vi "fade.vi"(8 "Brightness":dbl, 11 "In":u32) -> (3 "Out":u32)   [LabVIEW 2016]
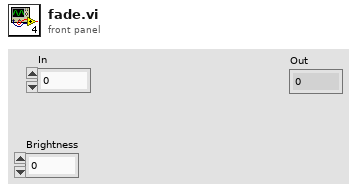
[diagram p1: front panel]
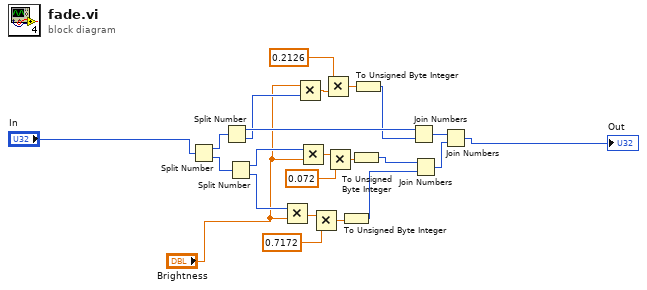
[diagram p0: block diagram]
diagram:
  n1 = Split Number(x="In") -> (hi(x)=w22:u16, lo(x)=w23:u16)
  n2 = Split Number(x=w22) -> (hi(x)=w20:u8, lo(x)=w13:u8)
  n3 = Split Number(x=w23) -> (hi(x)=w14:u8, lo(x)=w17:u8)
  n4 = Multiply(x=w17, y="Brightness") -> (x*y=w5:dbl)
  n5 = Multiply(x="Brightness", y=w13) -> (x*y=w9:dbl)
  n6 = Multiply(x=w14, y="Brightness") -> (x*y=w7:dbl)
  n7 = Multiply(x=w5, y=0.7172) -> (x*y=w4:dbl)
  n8 = Multiply(x=0.2126, y=w9) -> (x*y=w8:dbl)
  n9 = Multiply(x=w7, y=0.072) -> (x*y=w6:dbl)
  n10 = To Unsigned Byte Integer(number=w4) -> (unsigned 8bit integer=w16:u8)
  n11 = To Unsigned Byte Integer(number=w6) -> (unsigned 8bit integer=w15:u8)
  n12 = To Unsigned Byte Integer(number=w8) -> (unsigned 8bit integer=w12:u8)
  n13 = Join Numbers(hi=w20, lo=w12) -> ((hi.lo)=w21:u16)
  n14 = Join Numbers(hi=w15, lo=w16) -> ((hi.lo)=w10:u16)
  n15 = Join Numbers(hi=w21, lo=w10) -> ((hi.lo)=→"Out":u32)
